vi "1_1.vi"() -> ()   [LabVIEW 2023, in "2025.lvlib"]
uses:
  2025.lvlib
panel:
  out "Array 2":i32[](array[numeric])
  out "Numeric":i32
  in  "s":bool
  out "size(s)":i32
  in  "y":bool
  out "Array":i32[](array[numeric])
  out "Gauge":u8(knob) scale=0.0..100.0
  # "2666 too low"
  # "6707 too high"
  # "6248 too low"
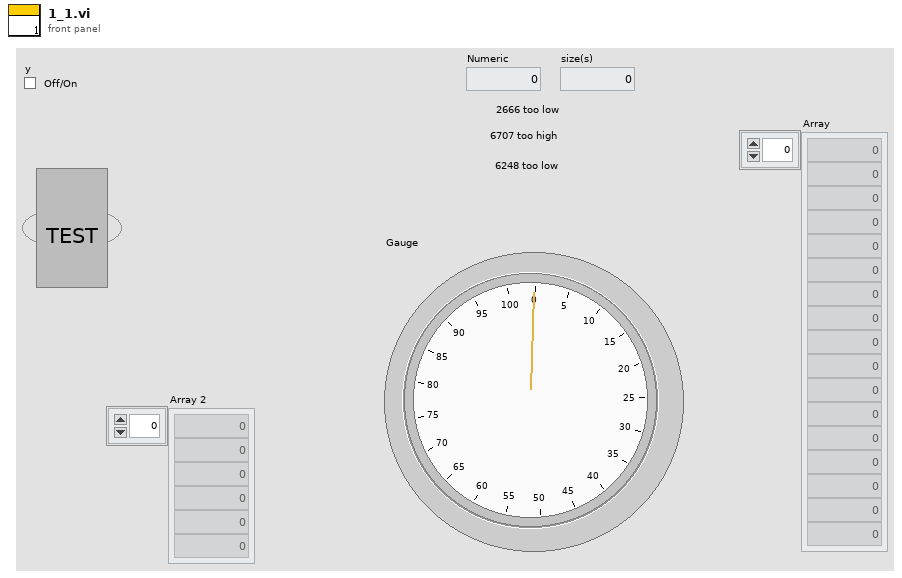
[diagram p1: front panel]
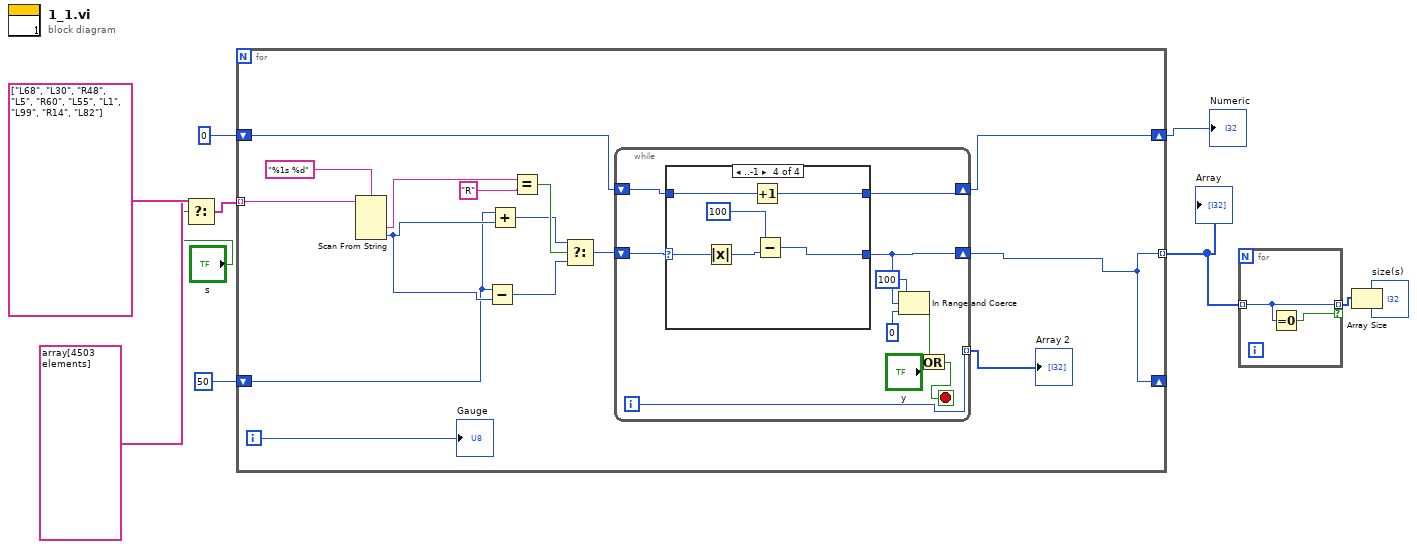
[diagram p0: block diagram]
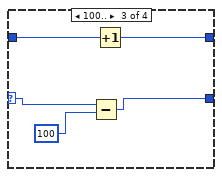
[diagram p4: hidden frame]
diagram:
  n1 = Select(t=string[] array[4503 elements], s="s", f=string[] ["L68", "L30", "R48", "L5", "R60", "L55", "L1", "L99", "R14", "L82"]) -> (s? t:f=w5:string[])
  n2 = for {
    tunnel: w5 -> [w24] mode=indexing
    shift-right: [w14] -> _
    shift-left: 50 -> [w16]
    tunnel: [w14] -> w8 mode=indexing
    shift-right: [w12] -> w1
    shift-left: 0 -> [w13]
    i -> [w25]
    n3 = Scan From String(format string="%1s %d", input string=w24) -> (output 1=w21:string, output 2=w22:i32)  [unwired: 4 in, 3 out]
    n4 = Subtract(x=w16, y=w22) -> (x-y=w17:i32)
    n5 = Add(x=w16, y=w22) -> (x+y=w18:i32)
    n6 = Equal?(x=w21, y="R") -> (x = y?=w19:bool)
    n7 = Select(t=w18, s=w19, f=w17) -> (s? t:f=w15:i32)
    n8 = while {
      shift-right: [w34] -> w14
      shift-left: w15 -> [w35]
      shift-right: [w27] -> w12
      shift-left: w13 -> [w28]
      tunnel: [w26] -> w11 mode=indexing
      i -> [w26]
      stop <- w30 stop-if-true
      n9 = case shown="..-1" w35 {
        selector: w35 -> [w37 w39 w44 w47]
        tunnel: [w37 w39 w42 w49] -> w34
        tunnel: [w36 w38 w40 w45] -> w27
        tunnel: w28 -> [w36 w38 w41 w46]
        frame 0 {
        }
        frame 1..99 {
        }
        frame 100.. {
          n10 = Subtract(x=w44, y=100) -> (x-y=w42:i32)
          n11 = Increment(x=w41) -> (x+1=w40:i32)
        }
        frame ..-1 {
          n12 = Absolute Value(x=w47) -> (abs(x)=w48:i32)
          n13 = Increment(x=w46) -> (x+1=w45:i32)
          n14 = Subtract(x=100 ("milliseconds to wait"), y=w48) -> (x-y=w49:i32)
        }
      }
      n15 = In Range and Coerce(upper limit=100, x=w34, lower limit=0) -> (In Range?=w31:bool)  [unwired: 1 out]
      n16 = Or(x=w31, y="y") -> (x .or. y?=w30:bool)
    }
    "Array 2" <- w11
    "Gauge" <- w25
  }
  "Array" <- w8
  "Numeric" <- w1
  n17 = for {
    tunnel: w8 -> [w52] mode=indexing
    tunnel: [w52] -> w7 mode=indexing if=w51
    n18 = Equal To 0?(x=w52) -> (x = 0?=w51:bool)
  }
  n19 = Array Size(array=w7) -> (size(s)=→"size(s)":i32)
